vi "2 LED Parallel Sequence.vi"(8 "Tag Name 2":string="Boolean processing result 0", 9 "Tag Name 1":string="Boolean processing result 0", 10 "Name":string="Led Sequence") -> (2 "Sequence out":refnum<class "Sequence Config.lvclass">)   [LabVIEW 2015, in "Sequencer Module tests.lvlib"]
uses:
  Sequencer Module tests.lvlib
  classes/Sequence Config/Sequence Config.lvclass
  classes/Wait Step Config/Wait Step Config.lvclass
  classes/Update Tag Step Config/Update Tag Configuration/Update Tag Config.lvclass
  <vilib>/NI/Tag Bus/tag/Data Type.ctl
  <vilib>/NI/Tag Bus Module Framework/channel/channel classification.ctl
  classes/Paralle Step Config/Parallel Step Config.lvclass
  <vilib>/NI/Tag Bus/tag/tag descriptor.lvclass
  <vilib>/NI/Tag Bus Module Framework/channel/TBM channel.lvclass
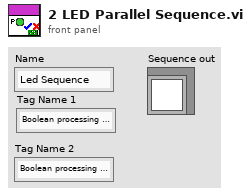
[diagram p1: front panel]
types:
  T1 = typedef "TBM channel.lvclass/channel classification.ctl" = enum16{"input data", "output data", "processing parameter", "processing result"}
  T2 = typedef "tag bus.lvlib/tag descriptor.lvclass/Data Type.ctl" = enum16{"Double", "Single", "I64", "I32", "I16", "I8", "U64", "U32", "U16", "U8", "Boolean", "String", "Array of Double", "Array of Single", "Array of I64", "Array of I32", "Array of I16", "Array of I8", "Array of U64", "Array of U32", "Array of U16", "Array of U8", "Array of Boolean", "Array of String"}
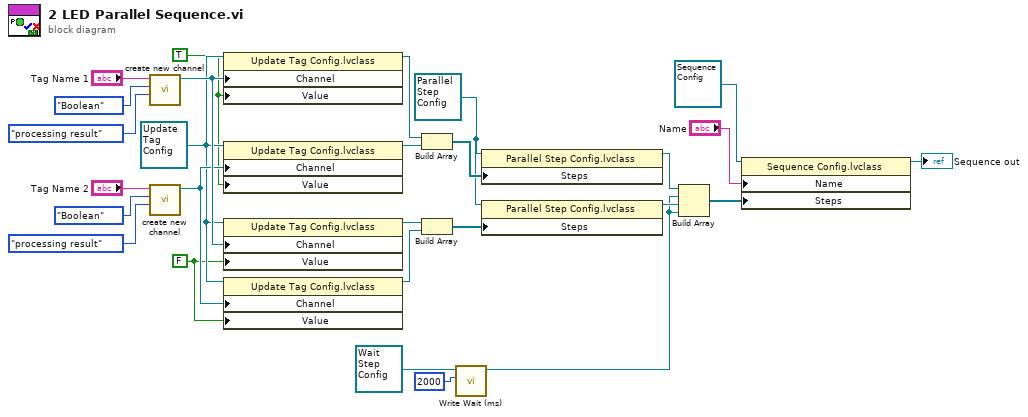
[diagram p0: block diagram]
diagram:
  w1 = refnum<class "Parallel Step Config.lvclass"> refnum ("Parallel Step Config.lvclass")
  w11 = FALSE
  w12 = TRUE
  w13 = refnum<class "Update Tag Config.lvclass"> refnum ("Update Tag Config.lvclass")
  n1 = call <vilib>:"create new channel.vi"("channel classification"=channel_classification."processing result", "data type"=Data_Type."Boolean" ("Data Type"), "channel name"="Tag Name 1") -> ("channel"=w18:refnum<class "TBM channel.lvclass">)  [unwired: 8 in]
  n2 = call <vilib>:"create new channel.vi"("channel classification"=channel_classification."processing result", "data type"=Data_Type."Boolean" ("Data Type"), "channel name"="Tag Name 2") -> ("channel"=w14:refnum<class "TBM channel.lvclass">)  [unwired: 8 in]
  n3 = property class="Update Tag Config.lvclass"(reference=w13, "Channel"=w18, "Value"=w12) -> (reference out=w10:refnum<class "Update Tag Config.lvclass">)  [unwired: 1 in, 1 out]
  n4 = property class="Update Tag Config.lvclass"(reference=w13, "Channel"=w14, "Value"=w12) -> (reference out=w9:refnum<class "Update Tag Config.lvclass">)  [unwired: 1 in, 1 out]
  n5 = property class="Update Tag Config.lvclass"(reference=w13, "Channel"=w18, "Value"=w11) -> (reference out=w5:refnum<class "Update Tag Config.lvclass">)  [unwired: 1 in, 1 out]
  n6 = property class="Update Tag Config.lvclass"(reference=w13, "Channel"=w14, "Value"=w11) -> (reference out=w4:refnum<class "Update Tag Config.lvclass">)  [unwired: 1 in, 1 out]
  n7 = Build Array(w10, w9) -> (w8:refnum<class "Update Tag Config.lvclass">[])
  n8 = Build Array(w5, w4) -> (w6:refnum<class "Update Tag Config.lvclass">[])
  n9 = call-dynamic "Write Wait (ms).vi"("Wait (ms)"=u32 2000, "Wait Step in"=refnum<class "Wait Step Config.lvclass"> refnum ("Wait Step Config.lvclass")) -> ("Wait Step out"=w2:refnum<class "Wait Step Config.lvclass">)  [unwired: 8 in, 1 out]
  n10 = property class="Parallel Step Config.lvclass"(reference=w1, "Steps"=w8) -> (reference out=w7:refnum<class "Parallel Step Config.lvclass">)  [unwired: 1 in, 1 out]
  n11 = property class="Parallel Step Config.lvclass"(reference=w1, "Steps"=w6) -> (reference out=w3:refnum<class "Parallel Step Config.lvclass">)  [unwired: 1 in, 1 out]
  n12 = Build Array(w7, w2, w3, w2) -> (w27:refnum<class "Step Config.lvclass">[])
  n13 = property class="Sequence Config.lvclass"(reference=refnum<class "Sequence Config.lvclass"> refnum ("Sequence Config.lvclass"), "Name"="Name", "Steps"=w27) -> (reference out=→"Sequence out":refnum<class "Sequence Config.lvclass">)  [unwired: 1 in, 1 out]
